vi "Calc Triangle Line Reciprocals.vi"(10 "Vertex 2":T1 {"UV"."v" min=0 max=1 step=0.1; "UV"."u" min=0 max=1 step=0.1}, 11 "Vertex 1":T1 {"UV"."v" min=0 max=1 step=0.1; "UV"."u" min=0 max=1 step=0.1}) -> (2 "Delta x":sgl, 3 "Starting x":sgl)   [LabVIEW 2022 SP3, in "Raster.lvlib"]
uses:
  Raster.lvlib
  3D/Vertex.ctl
  3D/Vector 3D.ctl
  UV.ctl
  3D/3D.lvlib
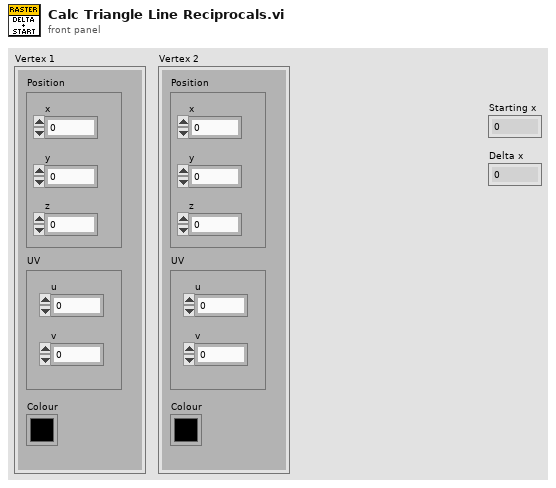
[diagram p1: front panel]
types:
  T1 = typedef "3D.lvlib/Vertex.ctl" = cluster{"Position":T2, "UV":T3, "Colour":u32}
  T2 = typedef "3D.lvlib/Vector 3D.ctl" = cluster{"x":sgl, "y":sgl, "z":sgl}
  T3 = typedef "Raster.lvlib/UV.ctl" = cluster{"u":sgl, "v":sgl}
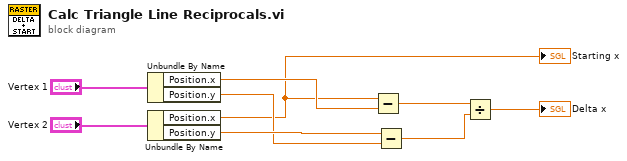
[diagram p0: block diagram]
diagram:
  n1 = Unbundle By Name("Vertex 1") -> ("Position.x"=w7:sgl, "Position.y"=w8:sgl)
  n2 = Unbundle By Name("Vertex 2") -> ("Position.x"=w4:sgl, "Position.y"=w9:sgl)
  "Starting x" <- w4
  n3 = Subtract(x=w4, y=w7) -> (x-y=w1:sgl)
  n4 = Subtract(x=w9, y=w8) -> (x-y=w2:sgl)
  n5 = Divide(x=w1, y=w2) -> (x/y=→"Delta x":sgl)
